vi "Exemple guider.vi"() -> ()   [LabVIEW 2018]
panel:
  out "Réponse":string
  in  "b":dbl
  in  "a":dbl
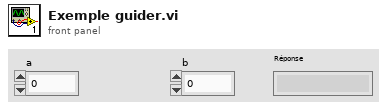
[diagram p1: front panel]
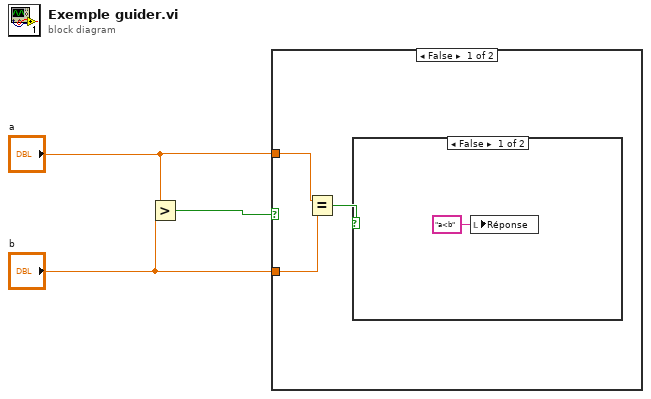
[diagram p0: block diagram]
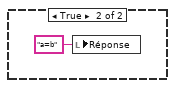
[diagram p2: hidden frame]
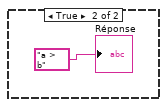
[diagram p3: hidden frame]
diagram:
  n1 = Greater?(x="a", y="b") -> (0:w3:bool)
  n2 = case shown="False" w3 {
    tunnel: "a" -> [w6 _]
    tunnel: "b" -> [w5 _]
    frame False {
      n3 = Equal?(x=w6, y=w5) -> (x = y?=w4:bool)
      n4 = case shown="False" w4 {
        frame False {
          n5 = local write "Réponse"("a<b" ("Réponse")) -> ()
        }
        frame True {
          n6 = local write "Réponse"("a=b" ("Réponse")) -> ()
        }
      }
    }
    frame True {
      "Réponse" <- "a > b" ("Réponse")
    }
  }
